vi "Sine out Amp.vi"(8 "error in (no error)":errorcluster, 10 "input 1":dbl, 11 "VISA Refnum in":refnum<visa-resource-name>) -> (0 "error out":errorcluster, 3 "VISA Refnum out":refnum<visa-resource-name>)   [LabVIEW 2025, in "MyLockIn.lvlib"]
uses:
  MyLockIn.lvlib
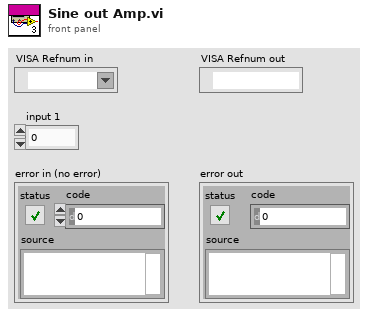
[diagram p1: front panel]
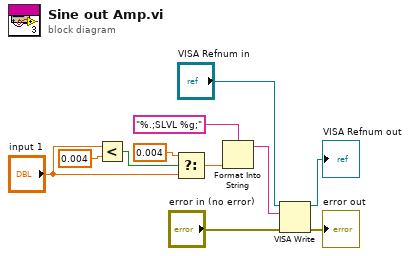
[diagram p0: block diagram]
diagram:
  n1 = Less?(x="input 1", y=0.004) -> (x < y?=w10:bool)
  n2 = Select(t=0.004, s=w10, f="input 1") -> (s? t:f=w11:dbl)
  n3 = Format Into String(format string="%.;SLVL %g;", w11) -> (resulting string=w3:string)  [unwired: 2 in, 1 out]
  n4 = VISA Write(VISA resource name="VISA Refnum in", write buffer=w3, error in (no error)="error in (no error)") -> (VISA resource name out=→"VISA Refnum out":refnum<visa-resource-name>, error out=→"error out":errorcluster)  [unwired: 1 out]
